vi "Accel Marker Update.vi"(6 "Marker Enum":T1, 7 "Listbox info":cluster{"InBounds":bool, "Row":i32}, 8 "error in (no error)":errorcluster, 9 "Select Active Row":bool, 10 "Marker Name":string, 11 "GUI in":refnum<class "GUI.lvclass">) -> (0 "error out":errorcluster, 3 "GUI out":refnum<class "GUI.lvclass">)   [LabVIEW 2020, in "GUI.lvlib" / "GUI.lvclass"]
uses:
  GUI.lvclass
  C:/Program Files/National Instruments/LabVIEW 2020/vi.lib/ActorFramework/Actor/Actor.lvclass
  Marker Enum.ctl
  GUI.lvclass/GUI.ctl
  <vilib>/ActorFramework/Actor/Actor.lvclass/Actor.ctl
  <vilib>/ActorFramework/Message Enqueuer/Message Enqueuer.lvclass/Message Enqueuer.ctl
  <vilib>/ActorFramework/Message Enqueuer/Init from Existing Queue.vi
  <vilib>/ActorFramework/Message Enqueuer/Message Enqueuer.lvclass
  <vilib>/ActorFramework/Actor/Actor.lvclass
  GUI Messages/Accel Marker Update Msg/Accel Marker Update Msg.lvclass
  Logging Messages/Markers Update Msg/Markers Update Msg.lvclass
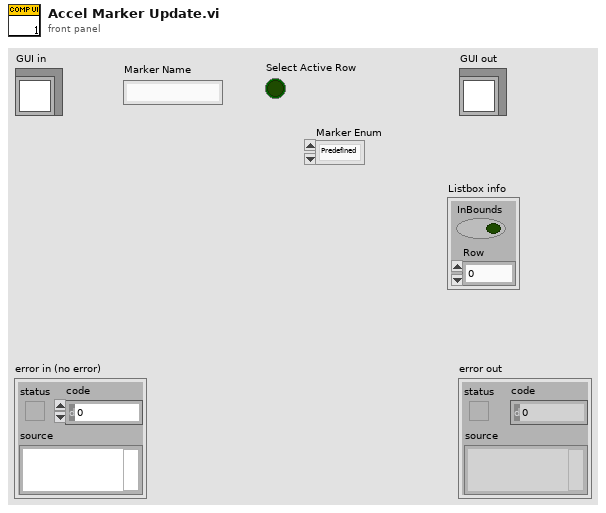
[diagram p1: front panel]
types:
  T1 = typedef "Marker Enum.ctl" = enum16{"Predefined", "Custom", "Delete Row", "Clear all"}
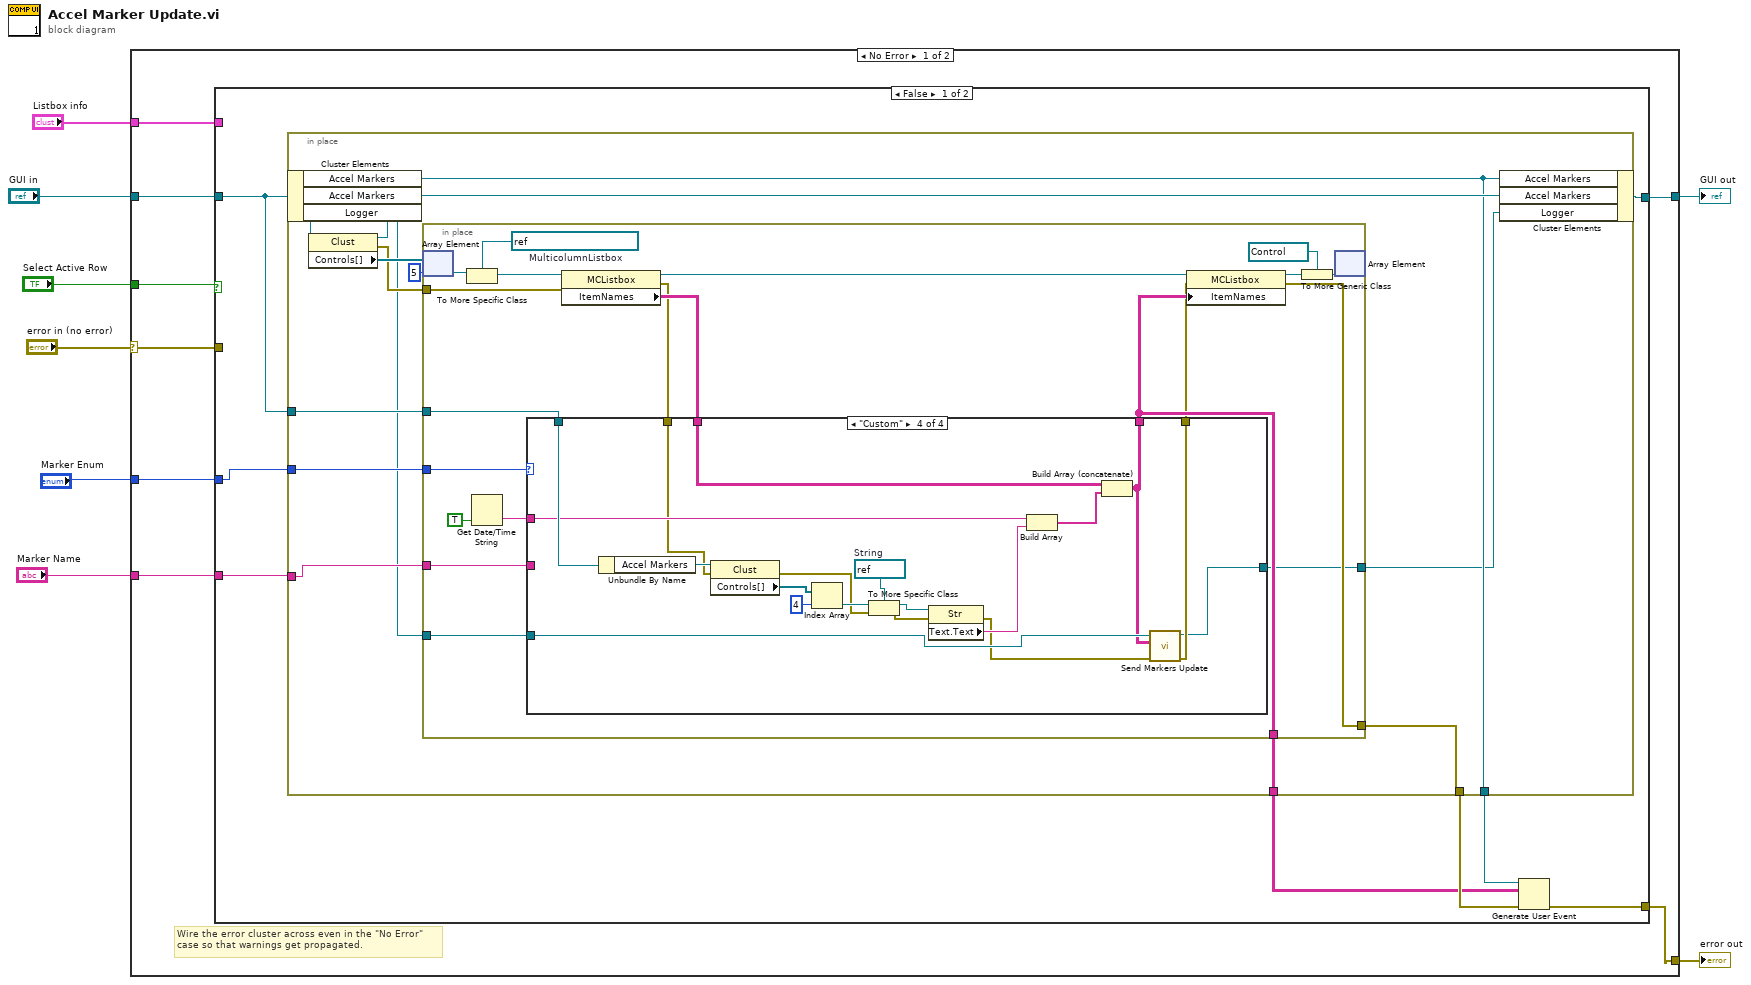
[diagram p0: block diagram]
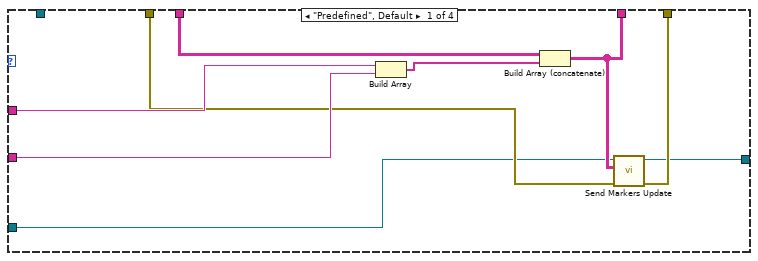
[diagram p2: hidden frame]
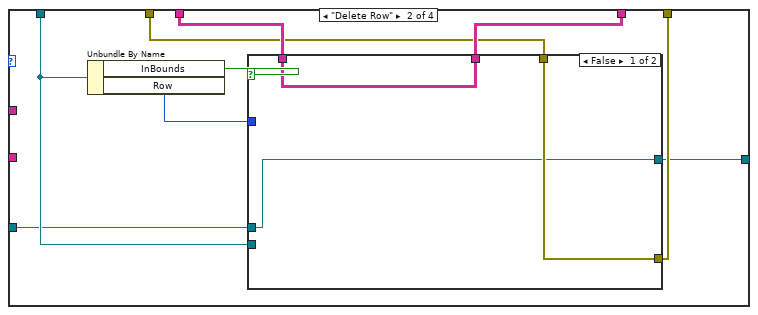
[diagram p3: hidden frame]
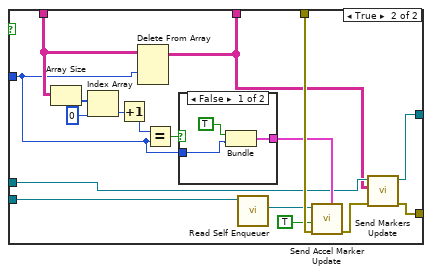
[diagram p4: hidden frame]
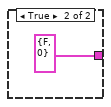
[diagram p5: hidden frame]
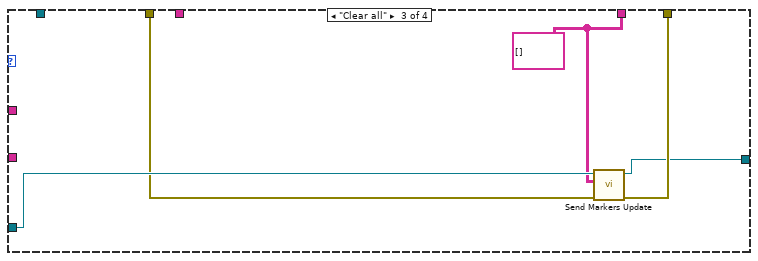
[diagram p6: hidden frame]
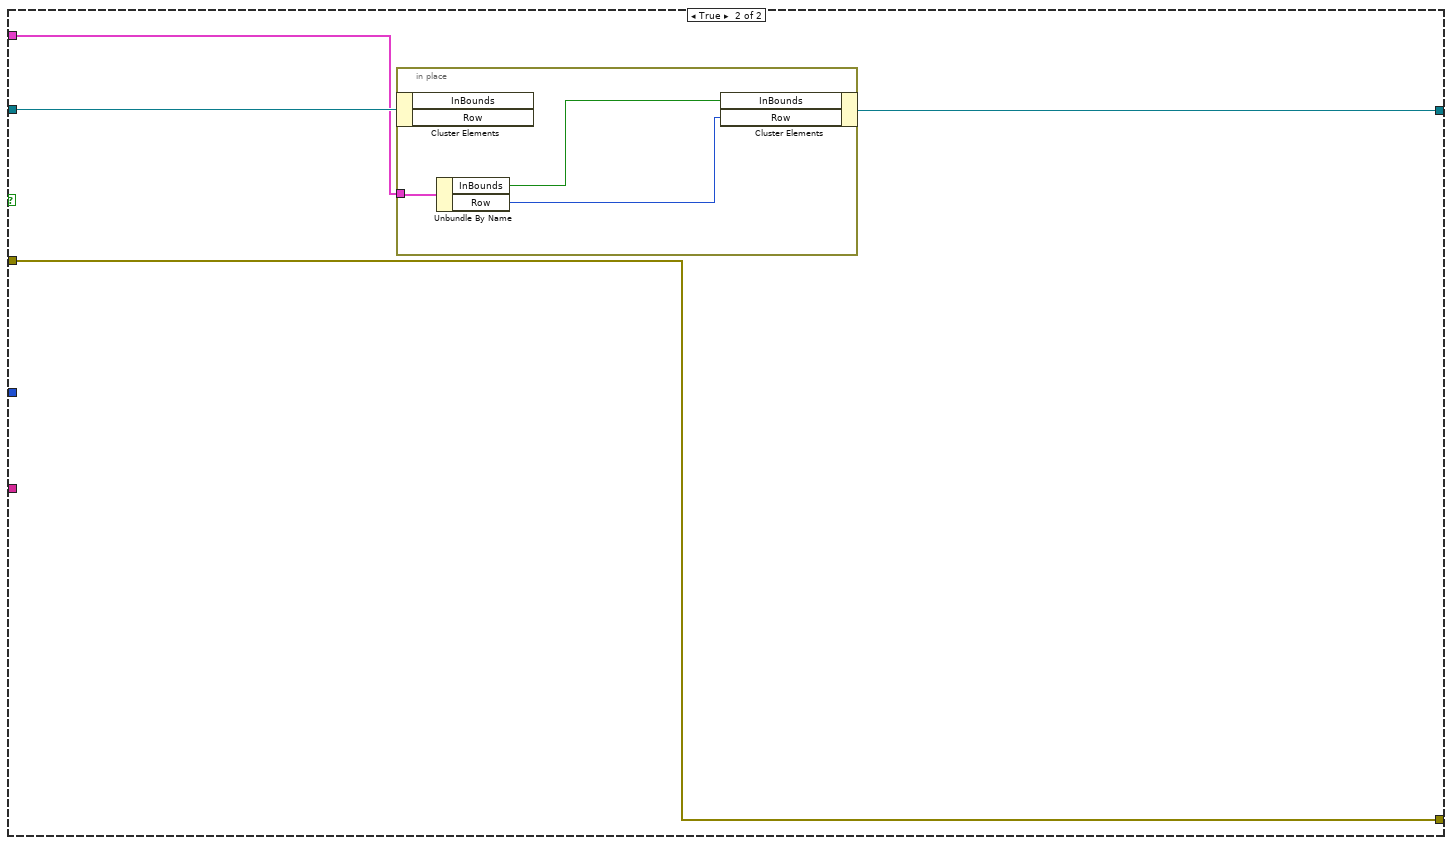
[diagram p7: hidden frame]
diagram:
  n1 = case shown="No Error" "error in (no error)" {
    selector: "error in (no error)" -> [w9 w132]
    tunnel: [w14 w132] -> w7
    tunnel: [w13 w131] -> w5
    tunnel: "GUI in" -> [w15 w131]
    tunnel: "Select Active Row" -> [w12 _]
    tunnel: "Marker Name" -> [w16 _]
    tunnel: "Marker Enum" -> [w11 _]
    tunnel: "Listbox info" -> [w10 _]
    frame No Error {
      # "Wire the error cluster across even in the \"No Error\"\ncase so that warnings get propagated."
      n2 = case shown="False" w12 {
        tunnel: w16 -> [w19 _]
        tunnel: w15 -> [w18 w127]
        tunnel: [w22 w124] -> w14
        tunnel: [w21 w125] -> w13
        tunnel: w11 -> [w20 _]
        tunnel: w10 -> [_ w126]
        tunnel: w9 -> [_ w124]
        frame False {
          n3 = in-place {
            in-place-border: [w32] -> w24
            in-place-border: [w31] -> w23
            in-place-border: w20 -> [w30]
            in-place-border: w19 -> [w29]
            in-place-border: w18 -> [w28]
            in-place-border: [w27] -> w17
            n4 = in-place-cluster #1(w18) -> ("Accel Markers"=w32:refnum<user-event>, "Accel Markers"=w37:refnum<vi>, "Logger"=w26:refnum<class "Message Enqueuer.lvclass">)
            n5 = property class="Clust"(reference=w37) -> (reference out=w34:refnum<vi>, error out=w33:errorcluster, "Controls[]"=w36:refnum<vi>[])  [unwired: 1 in]
            n6 = in-place {
              in-place-border: w33 -> [w50]
              in-place-border: [w49] -> w31
              in-place-border: w30 -> [w48]
              in-place-border: w29 -> [w47]
              in-place-border: w28 -> [w46]
              in-place-border: [w42] -> w27
              in-place-border: w26 -> [w39]
              in-place-border: [w38] -> w25
              w56 = refnum<vi> refnum  # MulticolumnListbox
              n7 = in-place-array #2(w36, 5) -> (w57:refnum<vi>)
              n8 = To More Specific Class(target class=w56, reference=w57) -> (specific class reference=w55:refnum<vi>)  [unwired: 1 in, 1 out]
              n9 = Get Date/Time String(want seconds? (F)=TRUE) -> (time string=w44:string)  [unwired: 2 in, 1 out]
              n10 = property class="MCListbox"(reference=w55, error in=w50) -> (reference out=w54:refnum<vi>, error out=w41:errorcluster, "ItemNames"=w43:string[][])
              n11 = case shown="\"Custom\"" w48 {
                tunnel: w47 -> [w65 _ _ _]
                tunnel: w44 -> [w66 _ _ w114]
                tunnel: w46 -> [_ w71 _ w123]
                tunnel: w43 -> [w64 w73 _ w111]
                tunnel: [w60 w72 w100 w107] -> w42
                tunnel: w41 -> [w62 w70 w103 w110]
                tunnel: [w61 w69 w102 w106] -> w40
                tunnel: w39 -> [w59 w68 w104 w109]
                tunnel: [w58 w67 w101 w105] -> w38
                frame "Predefined", Default {
                  n12 = Build Array(w66, w65) -> (w63:string[])
                  n13 = Build Array (concatenate)(w64, w63) -> (w60:string[][])
                  n14 = call "Send Markers Update.vi"("error in (no error)"=w62, "Accel Markers"=w60, "Message Enqueuer in"=w59) -> ("error out"=w61:errorcluster, "Message Enqueuer out"=w58:refnum<class "Message Enqueuer.lvclass">)  [unwired: 7 in]
                }
                frame "Delete Row" {
                  n15 = Unbundle By Name(w71) -> ("InBounds"=w75:bool, "Row"=w74:i32)
                  n16 = case shown="False" w75 {
                    tunnel: w74 -> [_ w84]
                    tunnel: w73 -> [w78 w91]
                    tunnel: [w78 w80] -> w72
                    tunnel: w71 -> [_ w95]
                    tunnel: w70 -> [w77 w94]
                    tunnel: [w77 w81] -> w69
                    tunnel: w68 -> [w76 w83]
                    tunnel: [w76 w79] -> w67
                    frame False {
                    }
                    frame True {
                      n17 = Array Size(array=w91) -> (size(s)=w90:i32[])
                      n18 = Index Array(array=w90, index=0) -> (element=w87:i32)
                      n19 = Increment(x=w87) -> (x+1=w86:i32)
                      n20 = Delete From Array(array=w91, index (row)=w84) -> (array with subset deleted=w80:string[][])  [unwired: 2 in, 1 out]
                      n21 = Equal?(x=w86, y=w84) -> (x = y?=w88:bool)
                      n22 = case shown="False" w88 {
                        tunnel: [w98 cluster{"InBounds":bool, "Row":i32} {"InBounds"=FALSE, "Row"=0} ("Listbox info")] -> w85
                        tunnel: w84 -> [w96 _]
                        frame False {
                          n23 = Bundle(TRUE, "Row"=w96) -> (w98:cluster{bool, "Row":i32})  [unwired: 1 in]
                        }
                        frame True {
                        }
                      }
                      n24 = call <vilib>:"Read Self Enqueuer.vi"("Actor"=w95) -> ("Self Enqueuer"=w93:refnum<class "Message Enqueuer.lvclass">)  [unwired: 10 in]
                      n25 = call "Send Accel Marker Update.vi"("Listbox info"=w85, "error in (no error)"=w94, "Select Active Row"=TRUE, "Message Enqueuer in"=w93) -> ("error out"=w82:errorcluster)  [unwired: 6 in, 1 out]
                      n26 = call "Send Markers Update.vi"("error in (no error)"=w82, "Accel Markers"=w80, "Message Enqueuer in"=w83) -> ("error out"=w81:errorcluster, "Message Enqueuer out"=w79:refnum<class "Message Enqueuer.lvclass">)  [unwired: 7 in]
                    }
                  }
                }
                frame "Clear all" {
                  w100 = string[][] [] ("ItemNames")
                  n27 = call "Send Markers Update.vi"("error in (no error)"=w103, "Accel Markers"=w100, "Message Enqueuer in"=w104) -> ("error out"=w102:errorcluster, "Message Enqueuer out"=w101:refnum<class "Message Enqueuer.lvclass">)  [unwired: 7 in]
                }
                frame "Custom" {
                  w118 = refnum<vi> refnum  # String
                  n28 = Unbundle By Name(w123) -> ("Accel Markers"=w122:refnum<vi>)
                  n29 = property class="Clust"(reference=w122, error in=w110) -> (error out=w113:errorcluster, "Controls[]"=w121:refnum<vi>[])  [unwired: 1 out]
                  n30 = Index Array(array=w121, index=4) -> (element=w119:refnum<vi>)
                  n31 = To More Specific Class(target class=w118, reference=w119, error in=w113) -> (specific class reference=w117:refnum<vi>, error out=w116:errorcluster)
                  n32 = property class="Str"(reference=w117, error in=w116) -> (error out=w108:errorcluster, "Text.Text"=w115:string)  [unwired: 1 out]
                  n33 = Build Array(w114, w115) -> (w112:string[])
                  n34 = Build Array (concatenate)(w111, w112) -> (w107:string[][])
                  n35 = call "Send Markers Update.vi"("error in (no error)"=w108, "Accel Markers"=w107, "Message Enqueuer in"=w109) -> ("error out"=w106:errorcluster, "Message Enqueuer out"=w105:refnum<class "Message Enqueuer.lvclass">)  [unwired: 7 in]
                }
              }
              n36 = property class="MCListbox"(reference=w54, error in=w40, "ItemNames"=w42) -> (reference out=w53:refnum<vi>, error out=w49:errorcluster)
              n37 = To More Generic Class(target class=refnum<vi> refnum ("element"), reference=w53) -> (generic class reference=w51:refnum<vi>)
              n38 = in-place-array #2(w51) -> ()  [unwired: 2 out]
            }
            n39 = in-place-cluster #1("Accel Markers"=w32, "Accel Markers"=w34, "Logger"=w25) -> (w21:refnum<class "GUI.lvclass">)
          }
          n40 = Generate User Event(user event=w24, event data cluster=w17, error in=w23) -> (error out=w22:errorcluster)  [unwired: 1 in, 1 out]
        }
        frame True {
          n41 = in-place {
            in-place-border: w126 -> [w130]
            n42 = in-place-cluster #3(w127) -> ()  [unwired: 2 out]
            n43 = Unbundle By Name(w130) -> ("InBounds"=w129:bool, "Row"=w128:i32)
            n44 = in-place-cluster #3("InBounds"=w129, "Row"=w128) -> (w125:refnum<class "GUI.lvclass">)
          }
        }
      }
    }
    frame Error {
    }
  }
  "error out" <- w7
  "GUI out" <- w5
